vi "CODCr质控流程 (子VI).vi"(10 "CODCr量程切换":enum32{"H", "L", "AUTO"}(ring)=enum."AUTO", 11 "CODCr":bool) -> (2 "CODCr中断报警":bool, 3 "布尔":bool)   [LabVIEW 2016, in "质控单元.lvlib"]
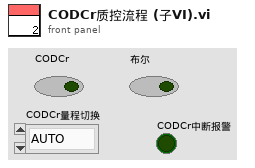
[diagram p1: front panel]
types:
  T1 = enum16{"待机", "启动水样测量", "水样测量中", "启动加标", "启动加标回收", "加标回收测量中", "结束"}
  T2 = cluster{"测量模式":enum16{"水样测量", "标样核查", "零点核查", "跨度核查", "空白测试", "加标回收", "平行样", "校零", "校标"}}
  T3 = enum16{"空闲", "水样测试", "标样核查", "零点核查", "跨度核查", "空白测试", "平行样测试", "加标回收", "空白校准", "标样校准", "初始化（清洗）"}
  T4 = cluster{"系统时间":timestamp, "工作状态":enum16{"空闲", "水样测试", "标样核查", "零点核查", "跨度核查", "空白测试", "平行样测试", "加标回收", "空白校准", "标样校准", "初始化（清洗）"}, "测量模式":enum16{"待机", "连续模式", "周期模式", "定点模式", "受控模式", "手动模式"}, "告警代码":enum16{"无告警", "缺试剂告警", "缺水样告警", "缺蒸馏水告警", "缺标液告警", "仪表漏液告警", "标定异常告警", "超量程告警", "加热异常", "低试剂预警", "超上限告警", "超下限告警", "仪表内部其他异常", "滴定异常告警", "电极异常告警", "量程切换告警", "参数设置告警", "PH电极电位异常", "电导率电极异常", "浊度光度异常", "溶解氧电极异常", "溶解氧光强异常", "温度异常告警", "PH异常告警", "溶解氧异常告警", "电导率异常告警", "浊度异常告警", "叶绿素异常告警", "藻密度异常告警", "蓝绿藻异常告警", "ORP异常告警", "氨氮异常告警", "清洁刷异常告警", "SD卡异常告警", "蓝牙异常告警", "Wifi异常告警", "流程异常告警"}, "故障代码":enum16{"无故障", "电机故障", "温度故障", "通讯故障", "滴定故障"}, "日志代码":u16, "软件版本":u16, "F0":sgl, "F1":sgl, "F2":sgl, "F3":sgl, "T":sgl, "H":sgl, "id":u16, "flowid":u16, "量程":u16, "总磷控温温度1":sgl, "营养盐控温温度2":sgl, "ADC":sgl}
  T5 = cluster{"因子编码":u32, "单位":u16, "标样参考值":sgl, "水样数据时间":timestamp, "水样实测值":sgl, "水样数据标识":string, "标样数据时间":timestamp, "标样实测值":sgl, "标样数据标识":string, "空白数据时间":timestamp, "空白实测值":sgl, "空白数据标识":string, "零点核查数据时间":timestamp, "零点核查实测值":sgl, "零点核查数据标识":string, "跨度核查数据时间":timestamp, "跨度核查实测值":sgl, "跨度核查数据标识":string, "加标回收数据时间":timestamp, "加标回收实测值":sgl, "加标回收数据标识":string, "平行样数据时间":timestamp, "平行样实测值":sgl, "平行样数据标识":string}
  T6 = cluster{"量程":dbl, "检出限":dbl, "加标前水样浓度":dbl, "加标后水样浓度":dbl, "加标水杯定容体积":dbl, "加标母液浓度":dbl, "加标体积":dbl, "加标回收率":dbl}
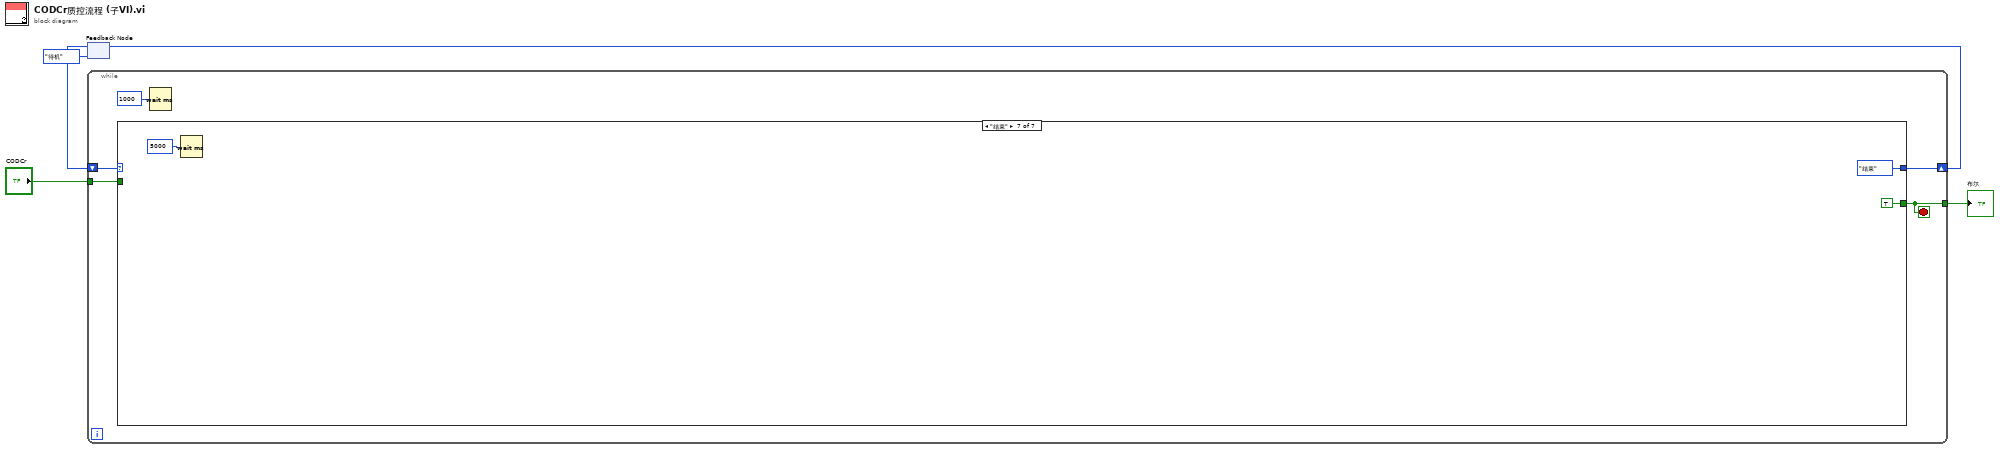
[diagram p0: block diagram]
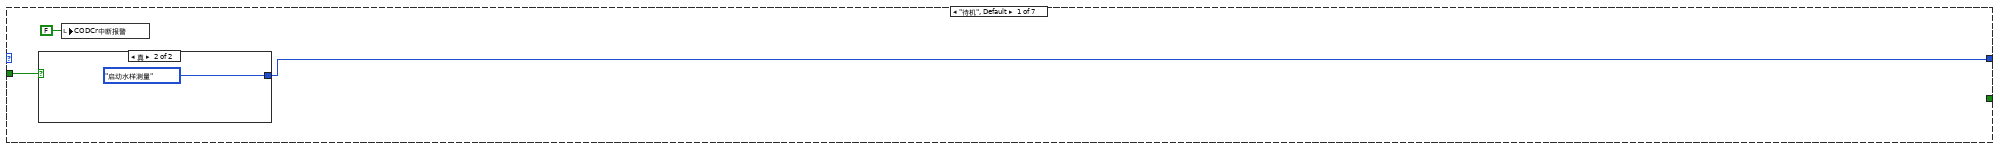
[diagram p2: hidden frame]
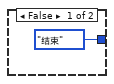
[diagram p3: hidden frame]
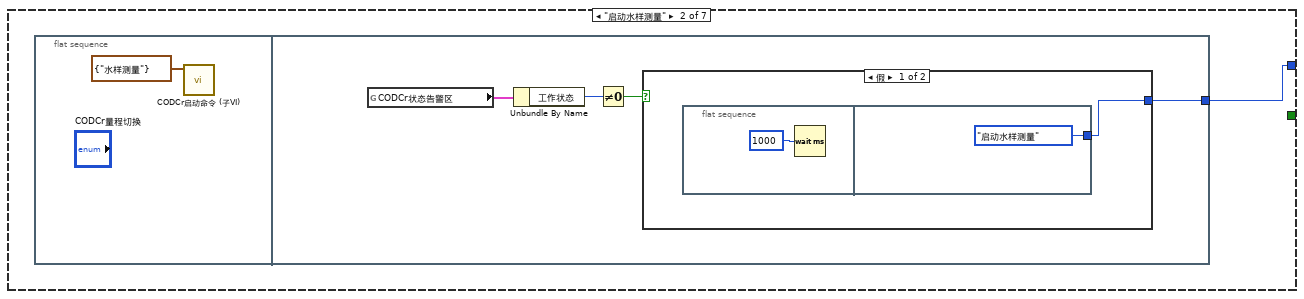
[diagram p4: hidden frame]
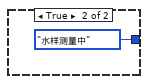
[diagram p5: hidden frame]
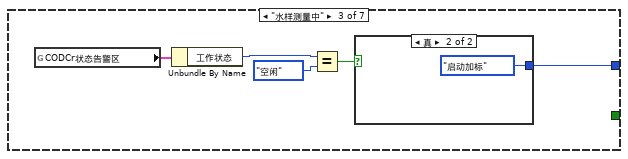
[diagram p6: hidden frame]
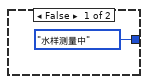
[diagram p7: hidden frame]
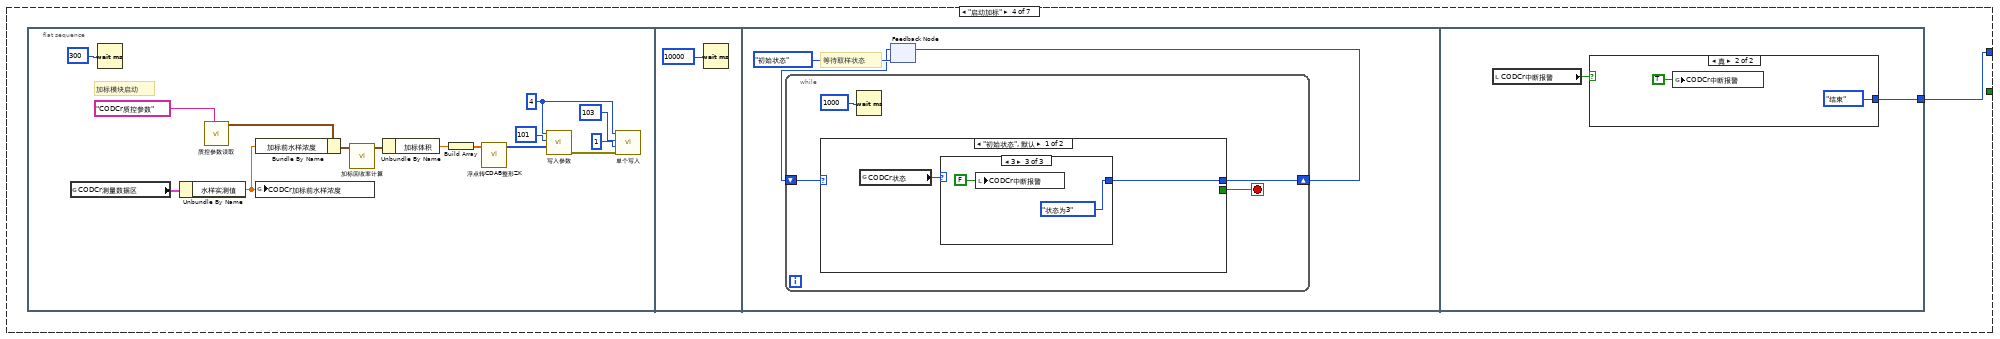
[diagram p8: hidden frame]
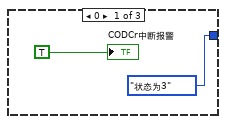
[diagram p9: hidden frame]
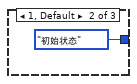
[diagram p10: hidden frame]
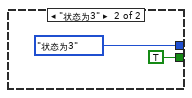
[diagram p11: hidden frame]
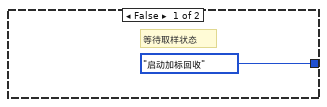
[diagram p12: hidden frame]
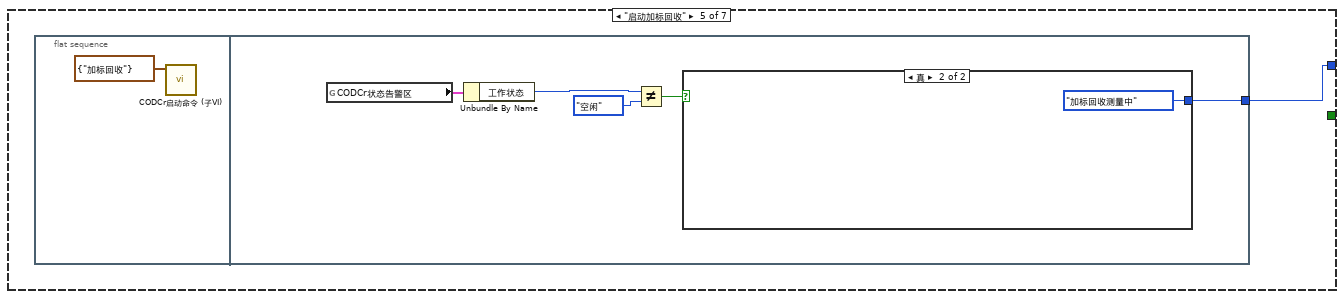
[diagram p13: hidden frame]
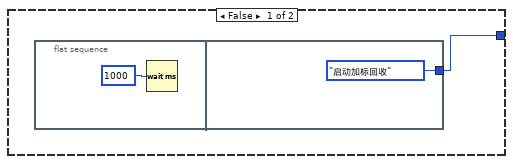
[diagram p14: hidden frame]
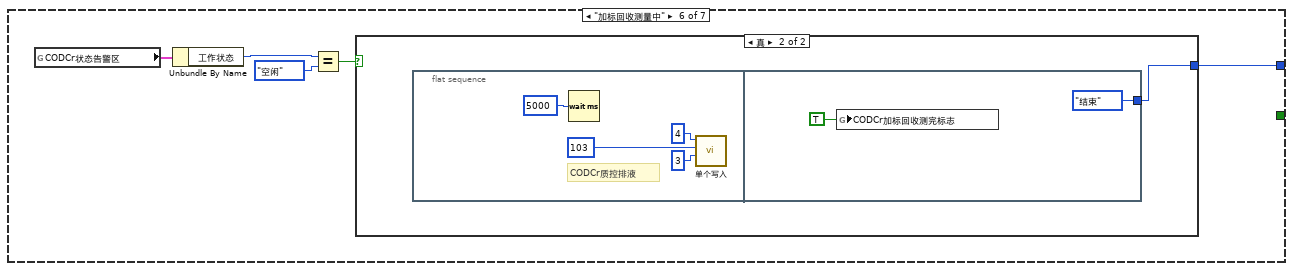
[diagram p15: hidden frame]
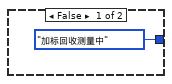
[diagram p16: hidden frame]
diagram:
  n1 = feedback #1(T1."待机") -> (w1:T1)
  n2 = while {
    tunnel: "CODCr" -> [w10]
    tunnel: [w8] -> w3
    shift-right: [w9] -> w4
    shift-left: w1 -> [w6]
    stop <- w8 stop-if-true
    n3 = case shown="\"结束\"" w6 {
      tunnel: [w13 w16 w30 w33 w71 w86 T1."结束"] -> w9
      tunnel: [_ _ _ _ _ _ TRUE] -> w8
      tunnel: w10 -> [w12 _ _ _ _ _ _]
      frame "待机", Default {
        n4 = case shown="真" w12 {
          tunnel: [T1."结束" T1."启动水样测量"] -> w13
          frame False {
          }
          frame True {
          }
        }
        n5 = local write "CODCr中断报警"(FALSE ("CODMn中断报警")) -> ()
      }
      frame "启动水样测量" {
        n6 = flat-sequence {
          tunnel: [w21] -> w16
          frame #0 {
            n7 = call "CODCr启动命令 (子VI).vi"("启动测量模式"=T2 {"测量模式"=enum."水样测量"}) -> ()  [unwired: 10 in, 1 out]
          }
          frame #1 {
            n8 = global read "与CODCr交互全局.vi" "CODCr状态告警区"() -> (w19:T4)
            n9 = Unbundle By Name(w19) -> ("工作状态"=w20:T3)
            n10 = Not Equal To 0?(x=w20) -> (x != 0?=w18:bool)
            n11 = case shown="假" w18 {
              tunnel: [w22 T1."水样测量中"] -> w21
              frame False {
                n12 = flat-sequence {
                  tunnel: [T1."启动水样测量"] -> w22
                  frame #0 {
                    n13 = Wait (ms)(milliseconds to wait=u32 1000 ("等待时间（毫秒）")) -> ()  [unwired: 1 out]
                  }
                  frame #1 {
                  }
                }
              }
              frame True {
              }
            }
          }
        }
      }
      frame "水样测量中" {
        n14 = global read "与CODCr交互全局.vi" "CODCr状态告警区"() -> (w27:T4)
        n15 = Unbundle By Name(w27) -> ("工作状态"=w26:T3)
        n16 = Equal?(x=w26, y=T3."空闲") -> (x = y?=w28:bool)
        n17 = case shown="真" w28 {
          tunnel: [T1."水样测量中" T1."启动加标"] -> w30
          frame False {
          }
          frame True {
          }
        }
      }
      frame "启动加标" {
        n18 = flat-sequence {
          tunnel: [w67] -> w33
          frame #0 {
            w37 = u16 4 ("value")
            # "加标模块启动"
            n19 = global read "与CODCr交互全局.vi" "CODCr测量数据区"() -> (w34:T5)
            n20 = Wait (ms)(milliseconds to wait=u32 300 ("等待时间（毫秒）")) -> ()  [unwired: 1 out]
            n21 = Unbundle By Name(w34) -> ("水样实测值"=w35:sgl)
            n22 = call "质控参数读取.vi"("section"="CODCr质控参数") -> ("参数"=w46:T6)  [unwired: 9 in, 1 out]
            n23 = Bundle By Name(cluster=w46, "加标前水样浓度"=w35) -> (w47:T6)
            n24 = global write "水样浓度全局.vi" "CODCr加标前水样浓度"(w35) -> ()
            n25 = call "加标回收率计算.vi"("参数"=w47) -> ("参数 out"=w45:T6)  [unwired: 10 in]
            n26 = Unbundle By Name(w45) -> ("加标体积"=w38:dbl)
            n27 = Build Array(w38) -> (w44:dbl[])
            n28 = call "浮点转CDAB整形ZK.vi"("浮点数"=w44) -> ("CDAB整形输出"=w39:u16[])  [unwired: 10 in]
            n29 = call "写入参数.vi"("values"=w39, "starting address"=u16 101, "Slave ID"=w37) -> ("error out"=w43:errorcluster)  [unwired: 8 in]
            n30 = call "单个写入.vi"("Error in"=w43, "value"=u16 1, "address"=u16 103, "Slave ID"=w37) -> ()  [unwired: 7 in, 1 out]
          }
          frame #1 {
            n31 = Wait (ms)(milliseconds to wait=u32 10000 ("等待时间（毫秒）")) -> ()  [unwired: 1 out]
          }
          frame #2 {
            # "等待取样状态"
            n32 = feedback #2(enum16{"初始状态", "状态为3"}."初始状态") -> (w51:enum16{"初始状态", "状态为3"})
            n33 = while {
              shift-right: [w55] -> w50
              shift-left: w51 -> [w56]
              stop <- w54 stop-if-true
              n34 = case shown="\"初始状态\", 默认" w56 {
                tunnel: [w58 enum16{"初始状态", "状态为3"}."状态为3"] -> w55
                tunnel: [_ TRUE] -> w54
                frame "初始状态", Default {
                  n35 = global read "加标回收状态全局变量.vi" "CODCr状态"() -> (w57:u16)
                  n36 = case shown="3" w57 {
                    tunnel: [enum16{"初始状态", "状态为3"}."状态为3" enum16{"初始状态", "状态为3"}."初始状态" enum16{"初始状态", "状态为3"}."状态为3"] -> w58
                    frame 0 {
                      "CODCr中断报警" <- TRUE ("CODMn中断报警")
                    }
                    frame 1, Default {
                    }
                    frame 3 {
                      n37 = local write "CODCr中断报警"(FALSE ("CODMn中断报警")) -> ()
                    }
                  }
                }
                frame "状态为3" {
                }
              }
              n38 = Wait (ms)(milliseconds to wait=u32 1000 ("等待时间（毫秒）")) -> ()  [unwired: 1 out]
            }
            n39 = feedback-in #2(w50) -> ()
          }
          frame #3 {
            n40 = local read "CODCr中断报警"() -> (w66:bool)
            n41 = case shown="真" w66 {
              tunnel: [T1."启动加标回收" T1."结束"] -> w67
              frame False {
                # "等待取样状态"
              }
              frame True {
                n42 = global write "质控中断报警全局.vi" "CODCr中断报警"(TRUE ("CODCr中断报警")) -> ()
              }
            }
          }
        }
      }
      frame "启动加标回收" {
        n43 = flat-sequence {
          tunnel: [w77] -> w71
          frame #0 {
            n44 = call "CODCr启动命令 (子VI).vi"("启动测量模式"=T2 {"测量模式"=enum."加标回收"}) -> ()  [unwired: 10 in, 1 out]
          }
          frame #1 {
            n45 = global read "与CODCr交互全局.vi" "CODCr状态告警区"() -> (w76:T4)
            n46 = Unbundle By Name(w76) -> ("工作状态"=w75:T3)
            n47 = Not Equal?(x=w75, y=T3."空闲") -> (x != y?=w73:bool)
            n48 = case shown="真" w73 {
              tunnel: [w78 T1."加标回收测量中"] -> w77
              frame False {
                n49 = flat-sequence {
                  tunnel: [T1."启动加标回收"] -> w78
                  frame #0 {
                    n50 = Wait (ms)(milliseconds to wait=u32 1000 ("等待时间（毫秒）")) -> ()  [unwired: 1 out]
                  }
                  frame #1 {
                  }
                }
              }
              frame True {
              }
            }
          }
        }
      }
      frame "加标回收测量中" {
        n51 = global read "与CODCr交互全局.vi" "CODCr状态告警区"() -> (w83:T4)
        n52 = Unbundle By Name(w83) -> ("工作状态"=w82:T3)
        n53 = Equal?(x=w82, y=T3."空闲") -> (x = y?=w84:bool)
        n54 = case shown="真" w84 {
          tunnel: [T1."加标回收测量中" w88] -> w86
          frame False {
          }
          frame True {
            n55 = flat-sequence {
              tunnel: [T1."结束"] -> w88
              frame #0 {
                # "CODCr质控排液"
                n56 = Wait (ms)(milliseconds to wait=u32 5000 ("等待时间（毫秒）")) -> ()  [unwired: 1 out]
                n57 = call "单个写入.vi"("value"=u16 3, "address"=u16 103, "Slave ID"=u8 4) -> ()  [unwired: 8 in, 1 out]
              }
              frame #1 {
                n58 = global write "质控测完标志全局 1.vi" "CODCr加标回收测完标志"(TRUE ("COD加标回收测完标志")) -> ()
              }
            }
          }
        }
      }
      frame "结束" {
        n59 = Wait (ms)(milliseconds to wait=u32 5000 ("等待时间（毫秒）")) -> ()  [unwired: 1 out]
      }
    }
    n60 = Wait (ms)(milliseconds to wait=u32 1000 ("等待时间（毫秒）")) -> ()  [unwired: 1 out]
  }
  "布尔" <- w3
  n61 = feedback-in #1(w4) -> ()
